vi "String_parse_try.vi"(11 "字符串":string="5.77\"}, \"op\": \"publish\"}{\"topic\": \"/chatter\", \"msg\": {\"data\": \"hello world 1479387235.87\"}, \"op\": \"publish\"}{\"topic\": \"/chatter\", \"msg\": {\"data\": \"hello world 1479387235.97\"}, \"op\": \"publish\"}{\"topic\": \"/chatter\", \"msg\": {\"data\": \"hello world 1479387236.07\"}, \"op\": \"publish\"}{\"topic\": \"/chatter\", \"msg\": {\"data\": \"hello world 1479387236.17\"}, \"op\": \"publish\"}{\"topic\": \"/chatter\", \"msg\": {\"data\": \"hello world 1479387236.27\"}, \"op\": \"publish\"}{\"topic\": \"/chatter\", \"msg\": {\"data\": \"hello world 14793") -> (2 "剩余字符串":string, 3 "data":string)   [LabVIEW 2014]
panel:
  out "值":cluster{"data":string}
  out "JSON out":string
  out "匹配之前的子字符串 2":string
  out "匹配+剩余字符串0":string
  out "匹配之前的子字符串":string
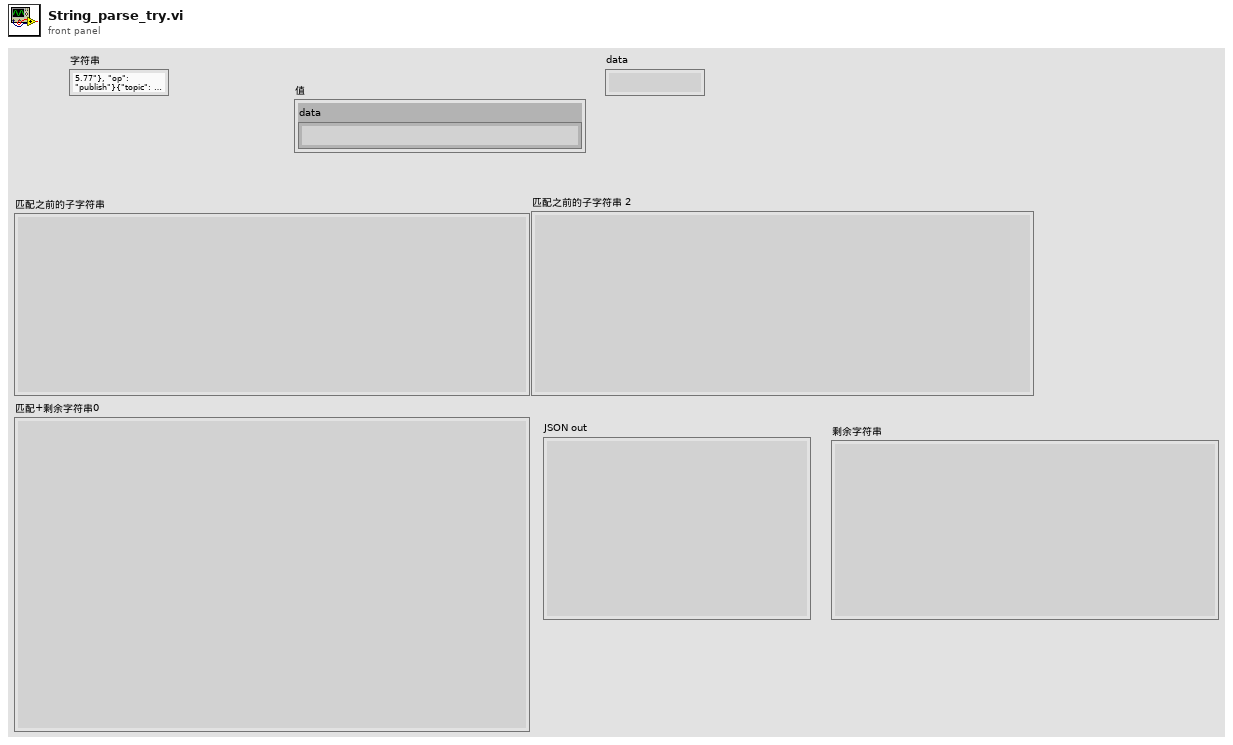
[diagram p1: front panel]
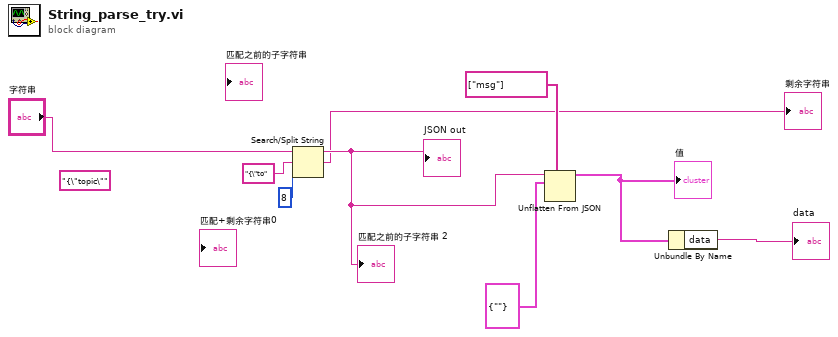
[diagram p0: block diagram]
diagram:
  (unwired) "{\"topic\"" ("搜索字符串")
  n1 = Search/Split String(string="字符串", search string/char (-)="{\"to" ("搜索字符串/字符(-)"), offset (0)=8 ("偏移量(0)")) -> (substring before match=w7:string, match + rest of string=→"剩余字符串":string)  [unwired: 1 out]
  "匹配之前的子字符串 2" <- w7
  "JSON out" <- w7
  n2 = Unflatten From JSON(path=string[] ["msg"] ("路径"), JSON string=w7, type and defaults=cluster{"data":string} {"data"=""} ("类型和默认值")) -> (value=w4:cluster{"data":string})  [unwired: 4 in, 1 out]
  "值" <- w4
  n3 = Unbundle By Name(w4) -> ("data"=→"data":string)
